vi "gm_sqlite_createtable.vi"(8 "error in (no error)":errorcluster, 11 "Database File":string) -> (0 "error out":errorcluster)   [LabVIEW 2011]
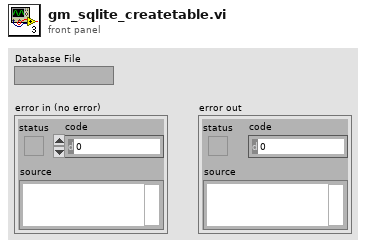
[diagram p1: front panel]
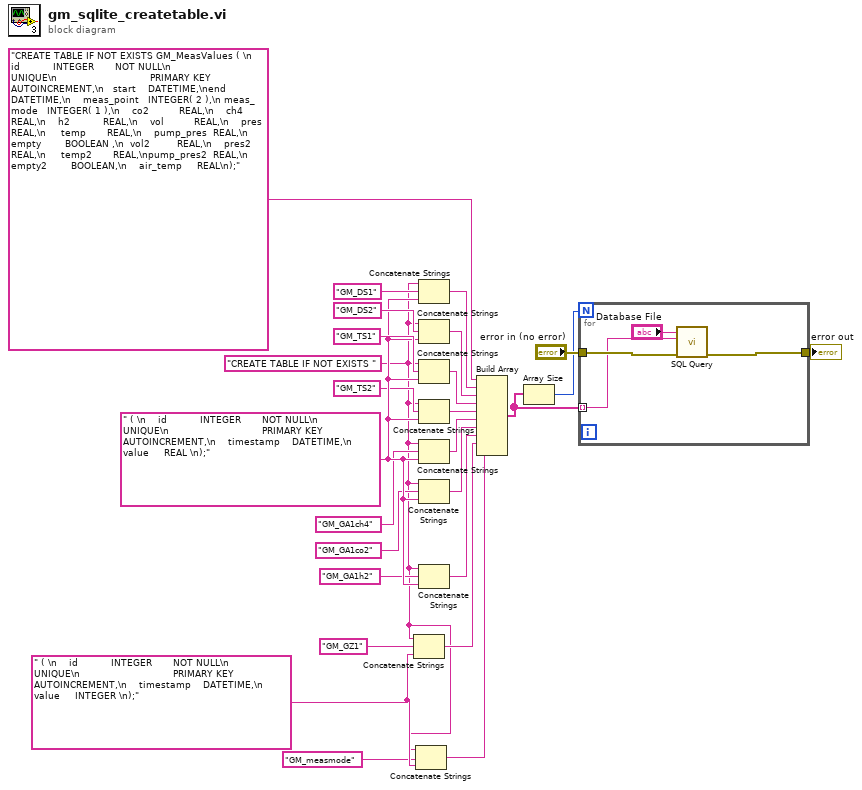
[diagram p0: block diagram]
diagram:
  w4 = " ( \n    id           INTEGER       NOT NULL\n                               UNIQUE\n                               PRIMARY KEY AUTOINCREMENT,\n    timestamp    DATETIME,\n    value     INTEGER \n);" ("SQL Query")
  w14 = " ( \n    id           INTEGER       NOT NULL\n                               UNIQUE\n                               PRIMARY KEY AUTOINCREMENT,\n    timestamp    DATETIME,\n    value     REAL \n);" ("SQL Query")
  w3 = "CREATE TABLE IF NOT EXISTS " ("SQL Query")
  n1 = Concatenate Strings(w3, "GM_GZ1" ("SQL Query"), w4) -> (w5:string)
  n2 = Concatenate Strings(w3, "GM_measmode" ("SQL Query"), w4) -> (w2:string)
  n3 = Concatenate Strings(w3, "GM_DS1" ("SQL Query"), w14) -> (w21:string)
  n4 = Concatenate Strings(w3, "GM_DS2" ("SQL Query"), w14) -> (w19:string)
  n5 = Concatenate Strings(w3, "GM_TS1" ("SQL Query"), w14) -> (w16:string)
  n6 = Concatenate Strings(w3, "GM_TS2" ("SQL Query"), w14) -> (w15:string)
  n7 = Concatenate Strings(w3, "GM_GA1ch4" ("SQL Query"), w14) -> (w11:string)
  n8 = Concatenate Strings(w3, "GM_GA1co2" ("SQL Query"), w14) -> (w10:string)
  n9 = Concatenate Strings(w3, "GM_GA1h2" ("SQL Query"), w14) -> (w9:string)
  n10 = Build Array("CREATE TABLE IF NOT EXISTS GM_MeasValues ( \n    id           INTEGER       NOT NULL\n                               UNIQUE\n                               PRIMARY KEY AUTOINCREMENT,\n   start    DATETIME,\nend    DATETIME,\n    meas_point   INTEGER( 2 ),\n meas_mode   INTEGER( 1 ),\n    co2          REAL,\n    ch4          REAL,\n    h2           REAL,\n    vol          REAL,\n    pres        REAL,\n     temp       REAL,\n    pump_pres  REAL,\n    empty        BOOLEAN ,\n  vol2         REAL,\n    pres2      REAL,\n     temp2       REAL,\npump_pres2  REAL,\n empty2        BOOLEAN,\n    air_temp     REAL\n);" ("SQL Query"), w21, w19, w16, w15, w11, w10, w9, w5, w2) -> (w23:string[])
  n11 = Array Size(array=w23) -> (size(s)=w24:i32)
  n12 = for {
    N: w24 -> [_]
    tunnel: "error in (no error)" -> [w30]
    tunnel: w23 -> [w29] mode=indexing
    tunnel: [w28] -> w22
    n13 = call "SQL Query.vi"("error in (no error)"=w30, "SQL Query"=w29, "Database File"="Database File") -> ("error out"=w28:errorcluster)  [unwired: 6 in, 2 out]
  }
  "error out" <- w22
